vi "CameraCtrl.vi"(6 "cam full size in":cluster{"xpixels":i32, "ypixels":i32}={"xpixels"=1024, "ypixels"=1024}, 8 "error constant":errorcluster, 10 "Camera Settings":T1={"EM Gain :"=100.0, "Pre Amp Gain :"=1.0, "VS Speed [Index] :"=1.0, "VS Amplitude :"=1.0, "Exposure Time [s] :"=1.0, "Temperature :"=0.2, "HS Speed [s]"=0.0, "Gain > 300 :"=FALSE}, 11 "Enum":enum16{"Start", "Stop", "Acquire", "Update"}(ring)) -> (0 "error constant 2":errorcluster, 2 "cam full size out":cluster{"xpixels":i32, "ypixels":i32}, 3 "Large Camera":i32[][](graph))   [LabVIEW 2019]
uses:
  CameraSettings.ctl
  <userlib>/atmcd32d.llb/ReadMode_mode typedef.ctl
  <userlib>/atmcd32d.llb/Error Code Enum typedef.ctl
panel:
  out "Camera connected":bool=TRUE
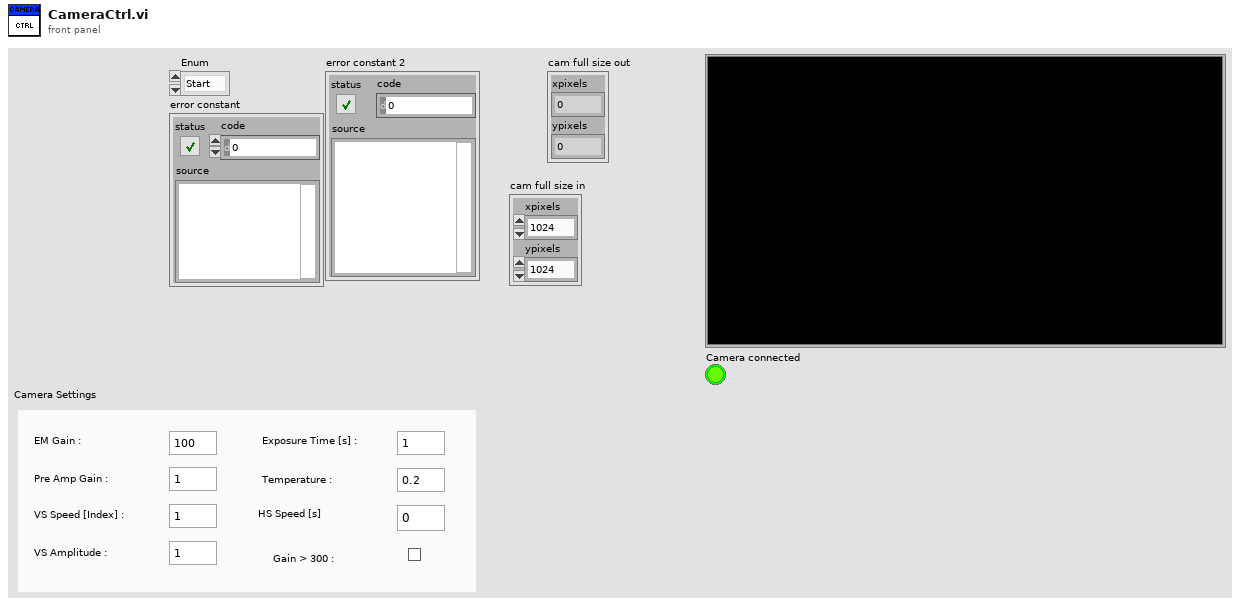
[diagram p1: front panel]
types:
  T1 = typedef "CameraSettings.ctl" = cluster{"EM Gain :":dbl, "Pre Amp Gain :":dbl, "VS Speed [Index] :":dbl, "VS Amplitude :":dbl, "Exposure Time [s] :":dbl, "Temperature :":dbl, "HS Speed [s]":dbl, "Gain > 300 :":bool}
  T2 = typedef "ReadMode_mode typedef.ctl" = enum16{"Full Vertical Binning", "Multi-Track", "Random-Track", "Single-Track", "Image"}
  T3 = cluster{"EM gain?":bool, "EM gain":u16, "preamp gain":enum16{"0", "1", "2", "3"}, "VS speed":enum16{"0", "1", "2", "3"}, "conv HS speed":enum16{"0", "1"}, "EM HS speed":enum16{"0", "1", "2", "3"}}
  T4 = typedef "Error Code Enum typedef.ctl" = enum32{"N/A (0)", "DRV_ERROR_CODES", "DRV_SUCCESS", "DRV_VXDNOTINSTALLED", "DRV_ERROR_SCAN", "DRV_ERROR_CHECK_SUM", "DRV_ERROR_FILELOAD", "DRV_UNKNOWN_FUNC", "DRV_ERROR_VXD_INIT", "DRV_ERROR_ADDRESS", "DRV_ERROR_PAGELOCK", "DRV_ERROR_PAGEUNLOCK", "DRV_ERROR_BOARDTEST", "DRV_ERROR_ACK", "DRV_ERROR_UP_FIFO", "DRV_ERROR_PATTERN", "N/A (16)", "DRV_ACQUISITION_ERRORS", "DRV_ACQ_BUFFER", "DRV_ACQ_DOWNFIFO_FULL", "DRV_PROC_UNKONWN_INSTRUCTION", "DRV_ILLEGAL_OP_CODE", "DRV_KINETIC_TIME_NOT_MET", "DRV_ACCUM_TIME_NOT_MET", "DRV_NO_NEW_DATA", "N/A (25)", "DRV_SPOOLERROR", "N/A (27)", "N/A (28)", "N/A (29)", "N/A (30)", "N/A (31)", "N/A (32)", "DRV_TEMPERATURE_CODES", "DRV_TEMPERATURE_OFF", "DRV_TEMPERATURE_NOT_STABILIZED", "DRV_TEMPERATURE_STABILIZED", "DRV_TEMPERATURE_NOT_REACHED", "DRV_TEMPERATURE_OUT_RANGE", "DRV_TEMPERATURE_NOT_SUPPORTED", "DRV_TEMPERATURE_DRIFT", "N/A (41)", "N/A (42)", "N/A (43)", "N/A (44)", "N/A (45)", "N/A (46)", "N/A (47)", "N/A (48)", "DRV_GENERAL_ERRORS", "DRV_INVALID_AUX", "DRV_COF_NOTLOADED", "DRV_FPGAPROG", "DRV_FLEXERROR", "DRV_GPIBERROR", "N/A (55)", "N/A (56)", "N/A (57)", "N/A (58)", "N/A (59)", "N/A (60)", "N/A (61)", "N/A (62)", "N/A (63)", "DRV_DATATYPE", "DRV_DRIVER_ERRORS", "DRV_P1INVALID", "DRV_P2INVALID", "DRV_P3INVALID", "DRV_P4INVALID", "DRV_INIERROR", "DRV_COFERROR", "DRV_ACQUIRING", "DRV_IDLE", "DRV_TEMPCYCLE", "DRV_NOT_INITIALIZED", "DRV_P5INVALID", "DRV_P6INVALID", "DRV_INVALID_MODE", "DRV_INVALID_FILTER", "DRV_I2CERRORS", "DRV_I2CDEVNOTFOUND", "DRV_I2CTIMEOUT", "DRV_P7INVALID", "N/A (84)", "N/A (85)", "N/A (86)", "N/A (87)", "N/A (88)", "N/A (89)", "DRV_IOCERROR", "DRV_VRMVERSIONERROR"}
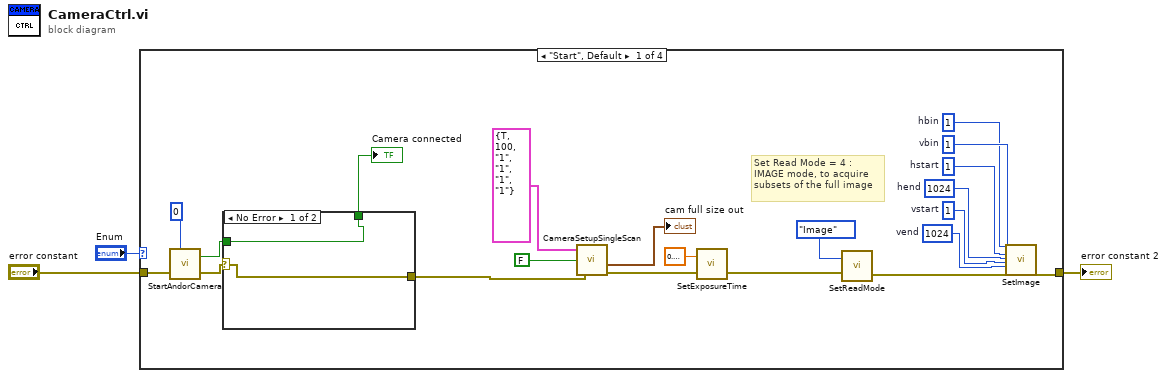
[diagram p0: block diagram]
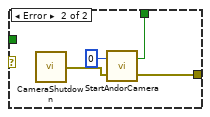
[diagram p2: hidden frame]
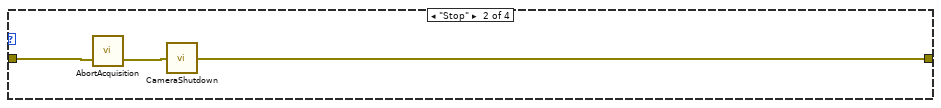
[diagram p3: hidden frame]
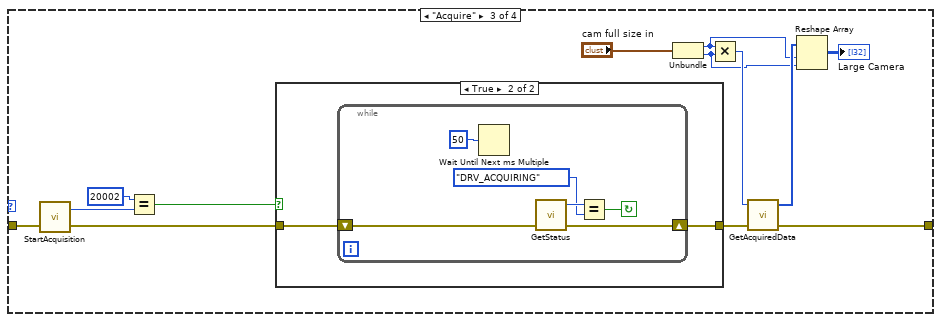
[diagram p4: hidden frame]
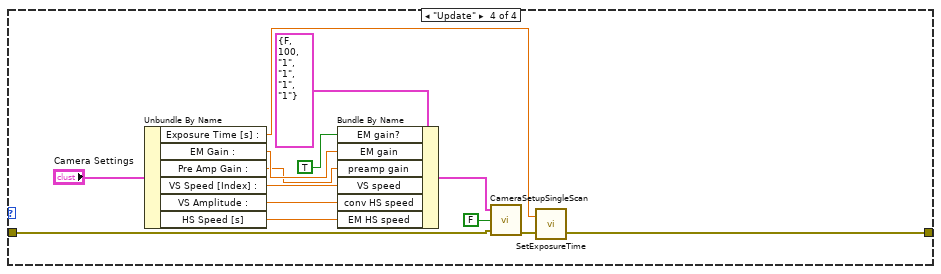
[diagram p6: hidden frame]
diagram:
  n1 = case shown="\"Start\", Default" "Enum" {
    tunnel: "error constant" -> [w23 w31 w46 w59]
    tunnel: [w8 w33 w40 w58] -> w1
    frame "Start", Default {
      w9 = 1024  # vend
      w10 = 1  # vstart
      w11 = 1024  # hend
      w12 = 1  # hstart
      w14 = 1  # vbin
      w13 = 1  # hbin
      # "Set Read Mode = 4 :\nIMAGE mode, to acquire\nsubsets of the full image"
      n2 = call "StartAndorCamera.vi"("error in (no error)"=w23, "Initial temp"=0) -> ("error out"=w7:errorcluster, "Camera OK?"=w5:bool)
      n3 = case shown="No Error" w7 {
        selector: w7 -> [w26 _]
        tunnel: [w26 w28] -> w4
        tunnel: [w25 w27] -> w6
        tunnel: w5 -> [w25 _]
        frame No Error {
        }
        frame Error {
          n4 = call "CameraShutdown.vi"() -> ("error out"=w30:errorcluster)  [unwired: 1 in]
          n5 = call "StartAndorCamera.vi"("error in (no error)"=w30, "Initial temp"=0) -> ("error out"=w28:errorcluster, "Camera OK?"=w27:bool)
        }
      }
      "Camera connected" <- w6
      n6 = call "CameraSetupSingleScan.vi"("error in (no error)"=w4, "EM adv"=FALSE, "Camera settings"=T3 {"EM gain?"=TRUE, "EM gain"=100, "preamp gain"=enum."1", "VS speed"=enum."1", "conv HS speed"=enum."1", "EM HS speed"=enum."1"}) -> ("error out"=w20:errorcluster, "image size"=→"cam full size out":cluster{"xpixels":i32, "ypixels":i32})  [unwired: 2 out]
      n7 = call <userlib>:"SetExposureTime.vi"("error in (no error)"=w20, "time"=sgl 0.1) -> ("error out"=w17:errorcluster)  [unwired: 1 out]
      n8 = call <userlib>:"SetReadMode.vi"("error in (no error)"=w17, "mode"=ReadMode_mode_typedef."Image") -> ("error out"=w15:errorcluster)  [unwired: 1 out]
      n9 = call <userlib>:"SetImage.vi"("hbin"=w13, "vbin"=w14, "hstart"=w12, "hend"=w11, "vstart"=w10, "vend"=w9, "error in (no error)"=w15) -> ("error out"=w8:errorcluster)  [unwired: 19 in, 1 out]
    }
    frame "Stop" {
      n10 = call <userlib>:"AbortAcquisition.vi"("error in (no error)"=w31) -> ("error out"=w32:errorcluster)  [unwired: 1 in, 1 out]
      n11 = call "CameraShutdown.vi"("error in (no error)"=w32) -> ("error out"=w33:errorcluster)
    }
    frame "Acquire" {
      n12 = call <userlib>:"StartAcquisition.vi"("error in (no error)"=w46) -> ("error out"=w42:errorcluster, "DLL error code"=w45:u32)  [unwired: 1 in]
      n13 = Equal?(x=u32 20002, y=w45) -> (x = y?=w43:bool)
      n14 = case shown="True" w43 {
        tunnel: w42 -> [w47 w49]
        tunnel: [w47 w48] -> w41
        frame False {
        }
        frame True {
          n15 = while {
            shift-right: [w54] -> w48
            shift-left: w49 -> [w55]
            stop <- w50 continue-if-true
            n16 = Wait Until Next ms Multiple(millisecond multiple=u32 50) -> ()  [unwired: 1 out]
            n17 = call <userlib>:"GetStatus.vi"("error in (no error)"=w55) -> ("error out"=w54:errorcluster, "status"=w53:T4)  [unwired: 2 in, 1 out]
            n18 = Equal?(x=w53, y=Error_Code_Enum_typedef."DRV_ACQUIRING") -> (x = y?=w50:bool)
          }
        }
      }
      n19 = Unbundle("cam full size in") -> ("xpixels"=w35:i32, "ypixels"=w34:i32)
      n20 = Multiply(x=w35, y=w34) -> (x*y=w39:i32)
      n21 = call <userlib>:"GetAcquiredData.vi"("error in (no error)"=w41, "size"=w39) -> ("error out"=w40:errorcluster, "array"=w38:i32[])  [unwired: 1 in, 1 out]
      n22 = Reshape Array(w38, w35, w34) -> (→"Large Camera":i32[][])
    }
    frame "Update" {
      n23 = Unbundle By Name("Camera Settings") -> ("Exposure Time [s] :"=w57:dbl, "EM Gain :"=w66:dbl, "Pre Amp Gain :"=w65:dbl, "VS Speed [Index] :"=w64:dbl, "VS Amplitude :"=w63:dbl, "HS Speed [s]"=w62:dbl)
      n24 = Bundle By Name(cluster=T3 {"EM gain?"=FALSE, "EM gain"=100, "preamp gain"=enum."1", "VS speed"=enum."1", "conv HS speed"=enum."1", "EM HS speed"=enum."1"} ("Camera settings"), "EM gain?"=TRUE, "EM gain"=w66, "preamp gain"=w65, "VS speed"=w64, "conv HS speed"=w63, "EM HS speed"=w62) -> (w69:T3)
      n25 = call "CameraSetupSingleScan.vi"("error in (no error)"=w59, "EM adv"=FALSE, "Camera settings"=w69) -> ("error out"=w60:errorcluster)  [unwired: 3 out]
      n26 = call <userlib>:"SetExposureTime.vi"("error in (no error)"=w60, "time"=w57) -> ("error out"=w58:errorcluster)  [unwired: 1 out]
    }
  }
  "error constant 2" <- w1
